vi "Pre Launch Init.vi"(11 "Test_Caller in":refnum<class "Test_Caller.lvclass">) -> (0 "error out":errorcluster, 3 "Test_Caller out":refnum<class "Test_Caller.lvclass">)   [LabVIEW 2025, in "Test_Caller.lvlib" / "Test_Caller.lvclass"]
doc: "<p>(<strong>Filename</strong>: <span class=\"dnl\">Actor Framework.lvlib:Actor.lvclass:Pre Launch Init.vi</span>)</p>\n<p>Defines behavior that occurs after the <a href=\"nihelplauncher://docs/csh?context=lvcore_lvcomm_af_launch_nested_actor\">Launch Nested Actor</a> method is invoked but before the actor's Actor Core method begins running.</p>\n<p>By default, this method does nothing. A descendant class may override it to define behavior.</p>"
uses:
  Test_Caller.lvclass
  <vilib>/ActorFramework/Actor/Actor.lvclass
  Test_Caller.lvclass/Test_Caller.ctl
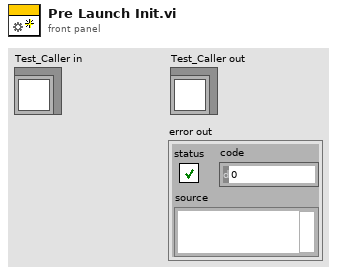
[diagram p1: front panel]
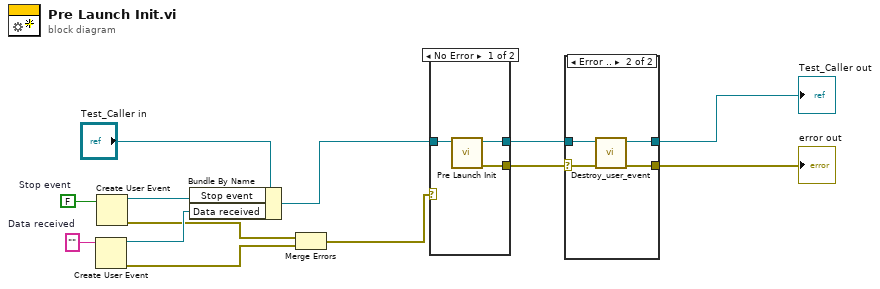
[diagram p0: block diagram]
diagram:
  w11 = ""  # Data received
  w12 = FALSE  # Stop event
  n1 = Create User Event(user event datatype=w11) -> (user event=w8:refnum<user-event>, error out=w5:errorcluster)  [unwired: 1 in]
  n2 = Create User Event(user event datatype=w12) -> (user event=w7:refnum<user-event>, error out=w4:errorcluster)  [unwired: 1 in]
  n3 = Bundle By Name(cluster="Test_Caller in", "Stop event"=w7, "Data received"=w8) -> (w9:refnum<class "Test_Caller.lvclass">)
  n4 = Merge Errors(w4, w5) -> (w6:errorcluster)
  n5 = case shown="No Error" w6 {
    selector: w6 -> [_ w17]
    tunnel: [w16 w17] -> w2
    tunnel: [w15 w18] -> w13
    tunnel: w9 -> [w14 w18]
    frame No Error {
      n6 = call-parent "Pre Launch Init.vi"("Actor in"=w14) -> ("error out"=w16:errorcluster, "Actor out"=w15:refnum<class "Test_Caller.lvclass">)  [unwired: 9 in]
    }
    frame Error {
    }
  }
  n7 = case shown="Error .." w2 {
    selector: w2 -> [w19 w21]
    tunnel: w13 -> [w20 w23]
    tunnel: [w20 w22] -> w3
    tunnel: [w19 w21] -> w1
    frame No Error {
    }
    frame Error {
      n8 = call "Destroy_user_event.vi"("Test_Caller in"=w23) -> ("Test_Caller out"=w22:refnum<class "Test_Caller.lvclass">)  [unwired: 9 in, 1 out]
    }
  }
  "error out" <- w1
  "Test_Caller out" <- w3
